vi "OKNstimTest.vi"() -> (0 "ComplexTest":T1, 1 "ComplexStim":T1, 2 "Stim":dbl[][](array[numeric]), 3 "Test":dbl[][](array[numeric]))   [LabVIEW 2016]
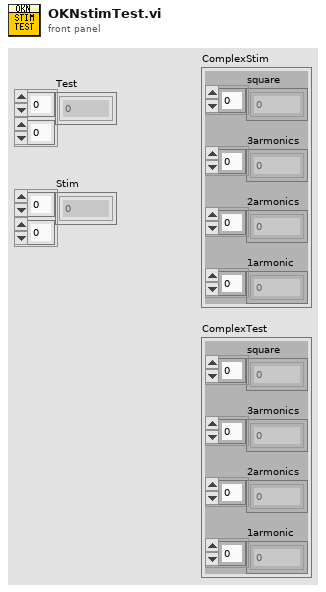
[diagram p1: front panel]
types:
  T1 = cluster{"square":dbl[], "3armonics":dbl[], "2armonics":dbl[], "1armonic":dbl[]}
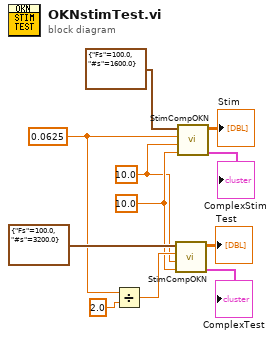
[diagram p0: block diagram]
diagram:
  w5 = 10.0 ("Offset")
  w4 = 10.0 ("Amp")
  w6 = 0.0625 ("frequency")
  n1 = Divide(x=w6, y=2.0) -> (x/y=w8:dbl)
  n2 = call "StimCompOKN.vi"("Offset"=w5, "Amp"=w4, "frequency"=w8, "sampling info"=cluster{"Fs":dbl, "#s":dbl} {"Fs"=100.0, "#s"=3200.0}) -> ("ComplexStim"=→"ComplexTest":T1, "Stim"=→"Test":dbl[][])  [unwired: 6 in]
  n3 = call "StimCompOKN.vi"("Offset"=w5, "Amp"=w4, "frequency"=w6, "sampling info"=cluster{"Fs":dbl, "#s":dbl} {"Fs"=100.0, "#s"=1600.0}) -> ("ComplexStim"=→"ComplexStim":T1, "Stim"=→"Stim":dbl[][])  [unwired: 6 in]
